vi "Wait for Windows Message.vi"(0 "win msg queue":T2, 1 "ms timeout (-1)":i32=-1, 2 "ignore previous (F)":bool, 3 "error in (no error)":errorcluster) -> (4 "Messages Remaining in Queue":i32, 5 "Sent":bool, 6 "win msg queue out":T2, 7 "Message":T1, 8 "timed out":bool, 9 "error out":errorcluster)   [LabVIEW 2017, in "Windows messages for Labview (32 and 64).lvlib"]
doc: "Asynchronously waits for the next windows message that is added to the queue and returns it. If ignore previous is set to true, all messages occurring before this wait are deleted. If it is set to false and prior messages are waiting in the queue, this VI returns immediately with the next message. No more than one Wait per queue should be active at any given time. Simultaneous waits on different queues are permissible.\n\nParameters:\nwin msq queue: the queue for which to wait.\n\nms timeout: timeout time in milliseconds\n\niqnore previous: whether to pay attention to messages added to the queue before this VI begins waiting. If true, only the message added to the queue while the VI is waiting are detected. All other prior messages are deleted. If false, if one or more messages are posted before the VI begins waiting, this VI returns immediately with the oldest message in the queue.\n\ntimed out: returns true if the timeout expired.\n\nMessage: the oldest message in the queue is removed and returned. (Usually this is the only message in the queue.) See Get Next Message.vi for more information.\n\nSent: returns true if the returned message was sent to the window (via SendMessage) or false if it was posted (via PostMessage). Note: messages that are sent will not have valid time or point parameters.\n\nMessage Remaining: the number of messsages still in the queue.\n\nErrors:\n6751: not a valid windows message queue.\n6752: no messages in queue when read was attempted."
uses:
  Windows messages for Labview (32 and 64).lvlib
  Win Msg Queue RefNum.ctl
  windows message x64.ctl
panel:
  in  "Occurrence RefNum":refnum<k4>
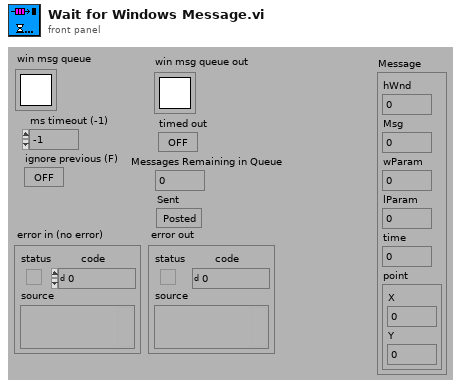
[diagram p1: front panel]
types:
  T1 = typedef "Windows messages for Labview (32 and 64).lvlib/windows message x64.ctl" = cluster{"hWnd":u64, "Msg":u32, "wParam":u64, "lParam":i32, "time":u32, "point":cluster{"X":i32, "Y":i32}}
  T2 = typedef "Windows messages for Labview (32 and 64).lvlib/Win Msg Queue RefNum.ctl" = refnum<k1>
  T3 = cluster{"hWnd":u32, "Msg":u32, "wParam":u32, "lParam":i32, "time":u32, "point":cluster{"X":i32, "Y":i32}}
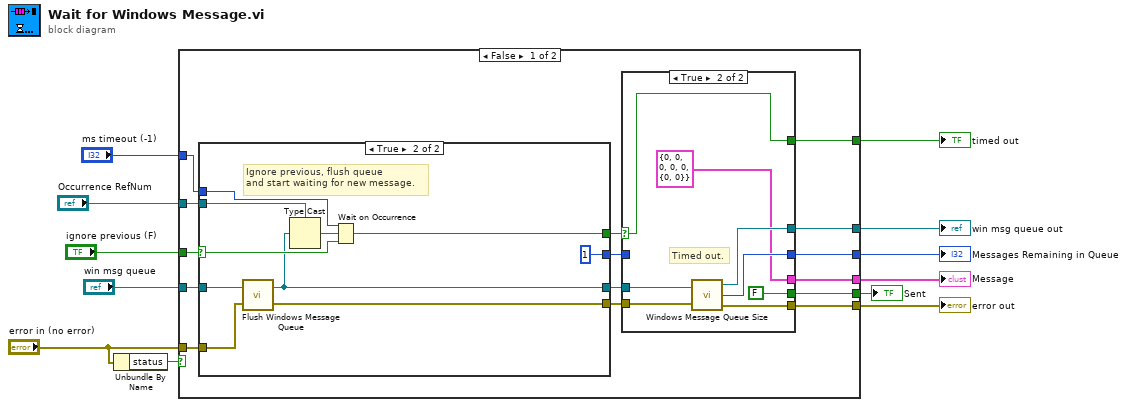
[diagram p0: block diagram]
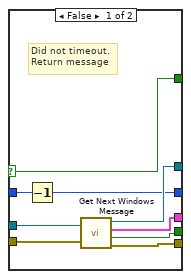
[diagram p2: hidden frame]
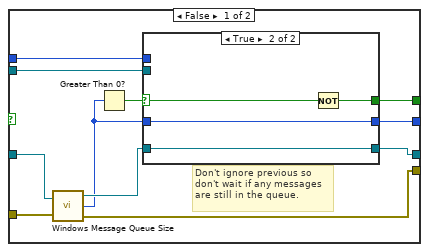
[diagram p3: hidden frame]
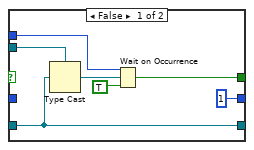
[diagram p4: hidden frame]
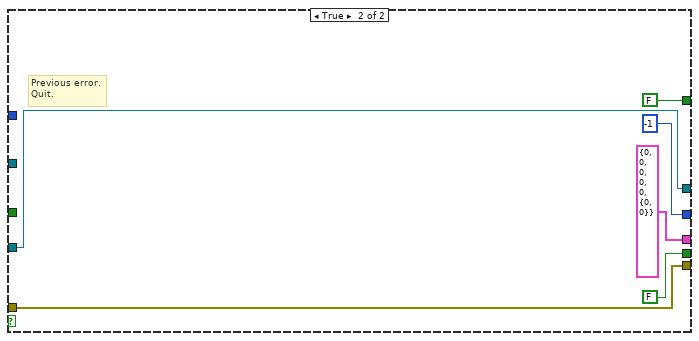
[diagram p5: hidden frame]
diagram:
  n1 = Unbundle By Name("error in (no error)") -> ("status"=w11:bool)
  n2 = case shown="False" w11 {
    tunnel: "error in (no error)" -> [w25 w81]
    tunnel: "win msg queue" -> [w26 w82]
    tunnel: "ms timeout (-1)" -> [w27 _]
    tunnel: "ignore previous (F)" -> [w24 _]
    tunnel: "Occurrence RefNum" -> [w23 _]
    tunnel: [w19 T3 {"hWnd"=0, "Msg"=0, "wParam"=0, "lParam"=0, "time"=0, "point"={"X"=0, "Y"=0}} ("Message")] -> w1
    tunnel: [w18 w82] -> w6
    tunnel: [w17 w81] -> w3
    tunnel: [w16 -1 ("Items in queue")] -> w4
    tunnel: [w15 FALSE] -> w5
    tunnel: [w13 FALSE ("Sent")] -> w2
    frame False {
      n3 = case shown="True" w24 {
        selector: w24 -> [_ w75]
        tunnel: w27 -> [w50 w74]
        tunnel: w26 -> [w55 w70]
        tunnel: w25 -> [w54 w71]
        tunnel: w23 -> [w53 w73]
        tunnel: [w49 w72] -> w22
        tunnel: [w48 w69] -> w21
        tunnel: [w47 w68] -> w20
        tunnel: [w45 1 ("Items in queue")] -> w14
        frame False {
          # "Don't ignore previous so\ndon't wait if any messages\nare still in the queue."
          n4 = call "Windows Message Queue Size.vi"("win msg queue"=w55, "error in (no error)"=w54) -> ("win msg queue out"=w51:T2, "Items in queue"=w46:i32, "error out"=w47:errorcluster)
          n5 = Greater Than 0?(x=w46) -> (x > 0?=w52:bool)
          n6 = case shown="True" w52 {
            selector: w52 -> [_ w66]
            tunnel: w53 -> [w61 _]
            tunnel: [w62 w64] -> w49
            tunnel: w51 -> [w58 w65]
            tunnel: w50 -> [w59 _]
            tunnel: [w58 w65] -> w48
            tunnel: w46 -> [_ w63]
            tunnel: [1 ("Items in queue") w63] -> w45
            frame False {
              n7 = Type Cast(type=w61, x=w58) -> (*(type *) &x=w60:refnum<k4>)
              n8 = Wait on Occurrence(1:TRUE, 2:w60, 3:w59) -> (0:w62:bool)
            }
            frame True {
              n9 = Not(x=w66) -> (.not. x?=w64:bool)
            }
          }
        }
        frame True {
          # "Ignore previous, flush queue\nand start waiting for new message."
          n10 = call "Flush Windows Message Queue.vi"("error in (no error)"=w71, "win msg queue"=w70) -> ("error out"=w68:errorcluster, "win msg queue out"=w69:T2)
          n11 = Type Cast(type=w73, x=w69) -> (*(type *) &x=w76:refnum<k4>)
          n12 = Wait on Occurrence(1:w75, 2:w76, 3:w74) -> (0:w72:bool)
        }
      }
      n13 = case shown="True" w22 {
        selector: w22 -> [w29 w39]
        tunnel: w21 -> [w36 w43]
        tunnel: w20 -> [w35 w44]
        tunnel: [w34 T1 {"hWnd"=0, "Msg"=0, "wParam"=0, "lParam"=0, "time"=0, "point"={"X"=0, "Y"=0}} ("Message 3")] -> w19
        tunnel: [w33 w42] -> w18
        tunnel: [w32 w41] -> w17
        tunnel: [w30 w40] -> w16
        tunnel: [w29 w39] -> w15
        tunnel: w14 -> [w31 _]
        tunnel: [w28 FALSE ("Sent")] -> w13
        frame False {
          # "Did not timeout.\nReturn message"
          n14 = Decrement(x=w31) -> (x-1=w30:i32)
          n15 = call "Get Next Windows Message.vi"("win msg queue"=w36, "error in (no error)"=w35) -> ("win msg queue out"=w33:T2, "Message"=w34:T1, "Sent"=w28:bool, "error out"=w32:errorcluster)
        }
        frame True {
          # "Timed out."
          n16 = call "Windows Message Queue Size.vi"("win msg queue"=w43, "error in (no error)"=w44) -> ("win msg queue out"=w42:T2, "Items in queue"=w40:i32, "error out"=w41:errorcluster)
        }
      }
    }
    frame True {
      # "Previous error.\nQuit."
    }
  }
  "error out" <- w3
  "timed out" <- w5
  "Messages Remaining in Queue" <- w4
  "win msg queue out" <- w6
  "Sent" <- w2
  "Message" <- w1
